vi "ProcessSensorData.vi"(8 "error in (no error)":errorcluster, 10 "clSensorData":T1, 11 "Class In":refnum<class "AnalysisPluginsBase.lvclass">) -> (0 "error out":errorcluster, 3 "Class Out":refnum<class "AnalysisPluginsBase.lvclass">)   [LabVIEW 2014, in "AnalysisPlugins.lvlib" / "AnalysisPluginsBase.lvclass"]
uses:
  AnalysisPluginsBase.lvclass
  Typedefs/clSensorData.ctl
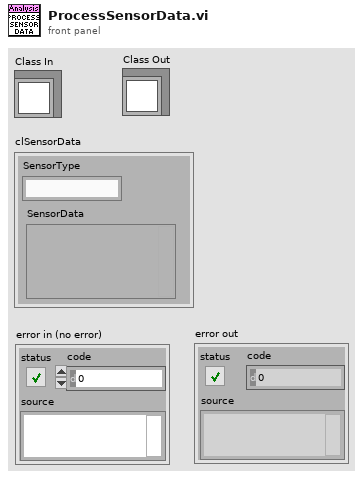
[diagram p1: front panel]
types:
  T1 = typedef "AnalysisPlugins.lvlib/AnalysisPluginsBase.lvclass/clSensorData.ctl" = cluster{"SensorType":string, "SensorData":variant}
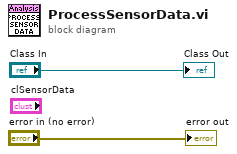
[diagram p0: block diagram]
diagram:
  "Class Out" <- "Class In"
  "error out" <- "error in (no error)"
